vi "Launcher.vi"() -> ()   [LabVIEW 2015]
panel:
  in  "Launch Process":bool
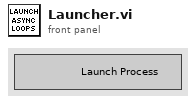
[diagram p1: front panel]
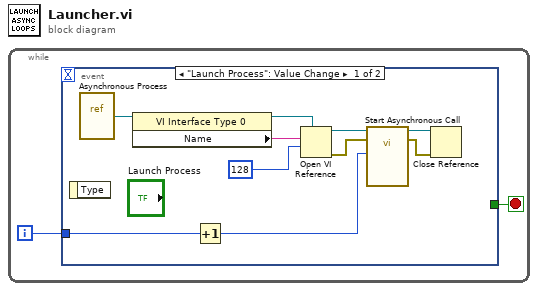
[diagram p0: block diagram]
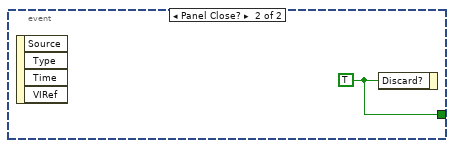
[diagram p2: hidden frame]
diagram:
  n1 = while {
    i -> [w1]
    stop <- w2 stop-if-true
    n2 = event shown="[0] \"Launch Process\": Value Change" {
      selector: _ -> [_ _]
      dyn-events: _ -> [_ _]
      timeout: _ -> [_ _]
      tunnel: [_ w13] -> w2
      tunnel: w1 -> [w4 _]
      event "Launch Process": Value Change {
        n3 = event-data() -> ()  [unwired: 1 in, 1 out]
        n4 = vi-ref "Asynchronous Process.vi"() -> (w10:refnum<vi>)
        n5 = property class="VI Interface Type 0"(reference=w10) -> (reference out=w11:refnum<vi>, "Name"=w9:string)  [unwired: 1 in, 1 out]
        n6 = Increment(x=w4) -> (x+1=w3:i32)
        n7 = Open VI Reference(type specifier VI Refnum (for type only)=w11, vi path=w9, options=128) -> (vi reference=w8:refnum<vi>, error out=w6:errorcluster)  [unwired: 3 in]
        n8 = call-by-ref "Start Asynchronous Call"(reference=w8, error in=w6, "Process"=w3) -> (reference out=w7:refnum<vi>, error out=w5:errorcluster)  [unwired: 11 in]
        n9 = Close Reference(reference=w7, error in (no error)=w5) -> ()  [unwired: 1 out]
      }
      event Panel Close? {
        w13 = TRUE ("Discard?")
        n10 = event-data() -> ()  [unwired: 1 in, 4 out]
        n11 = event-data("Discard?"=w13) -> ()  [unwired: 1 in, 1 out]
      }
    }
  }
